vi "MQTT_SSL_Disconnect.vi"(8 "error in (no error)":errorcluster, 11 "SSL_Connection":T1) -> (0 "error out":errorcluster)   [LabVIEW 2018, in "AWS_IoT.lvlib"]
doc: "Disconnects from an MQTT broker server.\n\n© 2015 - daq.io, LLC - Peter Adelhardt"
uses:
  AWS_IoT.lvlib
  Controls/SSL_Connection.ctl
  Controls/MessageType.ctl
  Controls/Retain_Flag.ctl
  Controls/QoS.ctl
  Controls/DUP_Flag.ctl
  Controls/Conn_FGV_Cmds.ctl
  Controls/Conn_Stat_FGV_Cmds.ctl
  Controls/Connection_Return_Codes.ctl
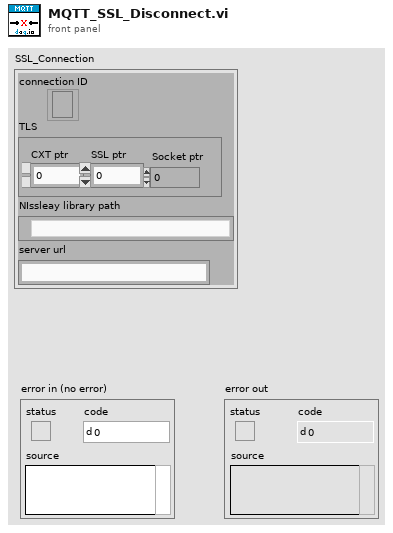
[diagram p1: front panel]
types:
  T1 = typedef "AWS_IoT.lvlib/SSL_Connection.ctl" = cluster{"connection ID":refnum<k5>, "TLS":cluster{"CXT ptr":i32, "SSL ptr":i32, "Socket ptr":i32}, "NIssleay library path":path, "server url":string}
  T2 = typedef "AWS_IoT.lvlib/Connection_Return_Codes.ctl" = enum16{"Connection accepted", "Connection refused: unacceptable protocol version", "Connection refused: identifier rejected", "Connection refused: Server unavailable", "Connection refused: bad user name or password", "Connection refused: not authorized"}
  T3 = typedef "AWS_IoT.lvlib/Conn_Stat_FGV_Cmds.ctl" = enum16{"Get", "Set"}
  T4 = typedef "AWS_IoT.lvlib/Conn_FGV_Cmds.ctl" = enum16{"Get", "Set", "Delete"}
  T5 = typedef "AWS_IoT.lvlib/DUP_Flag.ctl" = bool
  T6 = typedef "AWS_IoT.lvlib/QoS.ctl" = enum8{"At most once", "At least once", "Exactly once", "Reserved"}
  T7 = typedef "AWS_IoT.lvlib/Retain_Flag.ctl" = bool
  T8 = typedef "AWS_IoT.lvlib/MessageType.ctl" = enum32{"Reserved", "CONNECT", "CONNACK", "PUBLISH", "PUBACK", "PUBREC", "PUBREL", "PUBCOMP", "SUBSCRIBE", "SUBACK", "UNSUBSCRIBE", "UNSUBACK", "PINGREQ", "PINGRESP", "DISCONNECT", "Reserved2"}
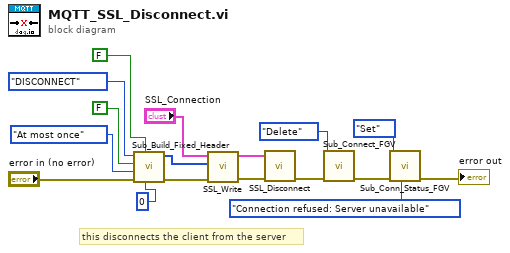
[diagram p0: block diagram]
diagram:
  # "this disconnects the client from the server"
  n1 = call "Sub_Build_Fixed_Header.vi"("Remaining Length"=u32 0, "Retain"=T7 FALSE, "error in (no error)"="error in (no error)", "QoS"=QoS."At most once", "DUP"=T5 FALSE, "MessageType"=MessageType."DISCONNECT") -> ("error out"=w11:errorcluster, "Fixed Header"=w10:u8[])  [unwired: 4 in]
  n2 = call "SSL_Write.vi"("error in (no error)"=w11, "data in"=w10, "SSL_Connection"="SSL_Connection") -> ("error out"=w9:errorcluster, "SSL_Connection"=w1:T1)  [unwired: 7 in]
  n3 = call "SSL_Disconnect.vi"("error in (no error)"=w9, "SSL_Connection"=w1) -> ("error out"=w8:errorcluster)  [unwired: 9 in]
  n4 = call "Sub_Connect_FGV.vi"("error in"=w8, "Command"=Conn_FGV_Cmds."Delete") -> ("error out"=w6:errorcluster)  [unwired: 8 in, 1 out]
  n5 = call "Sub_Conn_Status_FGV.vi"("Connection Status in"=Connection_Return_Codes."Connection refused: Server unavailable", "error in"=w6, "Command"=Conn_Stat_FGV_Cmds."Set") -> ("error out"=→"error out":errorcluster)  [unwired: 7 in, 1 out]
